vi "Lookup Executable Path.vi"(7 "Windows UTF8 Conversion":T1=enum."To OEM Code Page", 8 "error in":errorcluster, 11 "Executable Name":string) -> (0 "error out":errorcluster, 1 "Found":bool, 3 "Path":path)   [LabVIEW 2020, in "ase.lvlib" / "ase.lvclass"]
doc: "<B>Find the Full Path to the Executable by searching the System PATH.</B>\n\nIf the Executable is <B>not</B> found then the Path indicator will return <Not-A-Path>.\n\nOn Windows: The UTF8 converions mode can be set. On Linux this value is ignored."
uses:
  ase.lvclass
  Windows UTF8 Conversion Mode.ctl
  Error Internal Library Implementation Error.vi
  <vilib>/Utility/error.llb/Error Cluster From Error Code.vi
  ase.lvclass/ase.ctl
  bin/ase_32-3.dll
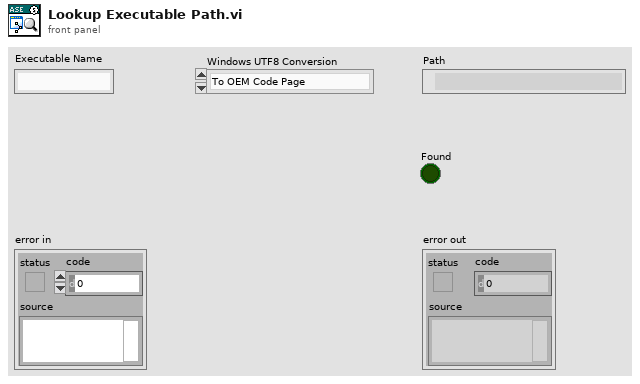
[diagram p1: front panel]
types:
  T1 = typedef "ase.lvlib/ase.lvclass/Windows UTF8 Conversion Mode.ctl" = enum8{"None (Pass Through UTF8)", "To ACP Code Page", "To OEM Code Page"}
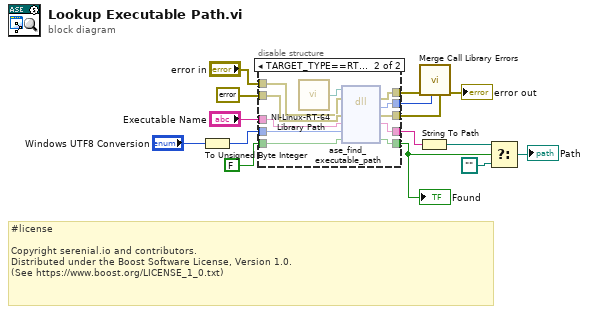
[diagram p0: block diagram]
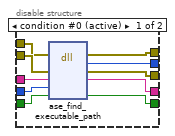
[diagram p2: hidden frame]
diagram:
  # "#license\n\nCopyright serenial.io and contributors.\nDistributed under the Boost Software License, Version 1.0.\n(See https://www.boost.org/LICENSE_1_0.txt)"
  n1 = To Unsigned Byte Integer(number="Windows UTF8 Conversion") -> (unsigned 8bit integer=w1:u8)
  n2 = disable-structure "Conditional Disable Structure" shown="TARGET_TYPE==RT&&OS==Linux" {
    disable-tunnel: errorcluster {"status"=FALSE, "code"=0, "source"=""} ("error") -> [w25 w36]
    disable-tunnel: FALSE -> [w24 w32]
    disable-tunnel: [w20 w27] -> w12
    disable-tunnel: [w21 w29] -> w11
    disable-tunnel: [w22 w28] -> w10
    disable-tunnel: [w23 w31] -> w9
    disable-tunnel: "Executable Name" -> [w19 w34]
    disable-tunnel: [w18 w30] -> w7
    disable-tunnel: "error in" -> [w17 w35]
    disable-tunnel: w1 -> [w16 w33]
    frame condition #0 (active) {
      n3 = dll-call lib="C:/serenial/lib/asynchronous-system-exec/LabVIEW/ase/ase/bin/ase_*-3.*" fn="ase_find_executable_path" ("AsyncSystemExec*.*:wrapperVersion")(error in=w17, "Error Out"=w25, "name"=w19, "conversion"=w16, "found"=w24) -> (error out=w20:errorcluster, "Error Code"=w21:i32, "Error Out"=w22:errorcluster, "name"=w18:string, "found"=w23:bool)  [unwired: 3 in, 1 out]
    }
    frame condition #1 {
      n4 = call "NI-Linux-RT-64 Library Path.vi"() -> ("Path"=w26:path)
      n5 = dll-call lib="?" fn="ase_find_executable_path" ("AsyncSystemExec*.*:wrapperVersion")(path in=w26, error in=w35, "Error Out"=w36, "name"=w34, "conversion"=w33, "found"=w32) -> (error out=w27:errorcluster, "Error Code"=w29:i32, "Error Out"=w28:errorcluster, "name"=w30:string, "found"=w31:bool)  [unwired: 2 in, 1 out]
    }
  }
  "Found" <- w9
  n6 = String To Path(string=w7) -> (path=w6:path)
  n7 = call "Merge Call Library Errors.vi"("Library Call Returned Error"=w10, "Error Code"=w11, "error in"=w12) -> ("error IO"=→"error out":errorcluster)  [unwired: 8 in]
  n8 = Select(t=w6, s=w9, f=path "" ("Not A Path Constant")) -> (s? t:f=→"Path":path)
